vi "Format when sending reply logger (SubVI).vi"(1 "sent message":string, 2 "status":string, 3 "queue name":string) -> (0 "info to log":string)   [LabVIEW 2016]
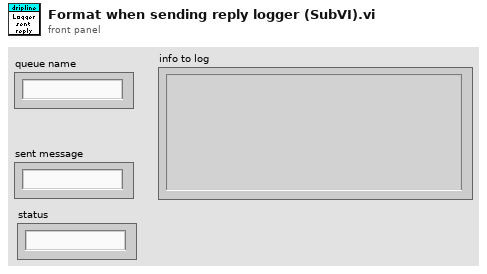
[diagram p1: front panel]
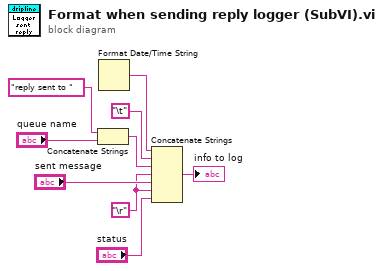
[diagram p0: block diagram]
diagram:
  w2 = "\r"
  n1 = Concatenate Strings("reply sent to " ("status"), "queue name") -> (w4:string)
  n2 = Format Date/Time String() -> (date/time string=w6:string)  [unwired: 3 in]
  n3 = Concatenate Strings(w6, "\t", w4, w2, "sent message", w2, "status") -> (→"info to log":string)
